vi "PSP-Nx-DM.vi"(0 "Cluster":cluster{"Button to Check":u16} {"Button to Check" items=["Start", "Select", "Up", "Down", "Left", "Right", "^", "[]", "X", "O", "L1", "L2", "L3", "R1", "R2", "R3"]}, 2 "NXT":T2={"error"={"status"=FALSE, "code"=0, "source"=""}, "address"="", "NXT #"=-1, "Show Error"=TRUE, "Connection"=4} {"Connection" items=["USB", "Bluetooth", "USB then Bluetooth", "Last Connection", "Preference"]}, 3 "Input Port":T3 items=["Port 1", "Port 2", "Port 3", "Port 4"]) -> (1 "output cluster":T1, 4 "NXT dup":T2={"error"={"status"=FALSE, "code"=0, "source"=""}, "address"="", "NXT #"=-1, "Show Error"=TRUE, "Connection"=4} {"Connection" items=["USB", "Bluetooth", "USB then Bluetooth", "Last Connection", "Preference"]})   [LabVIEW 2009]
uses:
  <vilib>/NXT/Block Support/NXT_InputPort.ctl
  <vilib>/NXT/Subs/LVHSConnector.ctl
  <vilib>/NXT/Block Support/HWPage.SensorType.ctl
  <vilib>/NXT/Block Support/HWPage.SensorMode.ctl
panel:
  # "mindsensors.com\nCopyright (c) 2009 by mindsensors.com\nEmail: info (<at>) mindsensors (<dot>) com\n\nThis program is free software. You can redistribute it and/or modify\nit under the terms of the GNU General Public License as published by\nthe Free Software Foundation; version 3 of the License.\nRead the license at: http://www.gnu.org/licenses/gpl.txt"
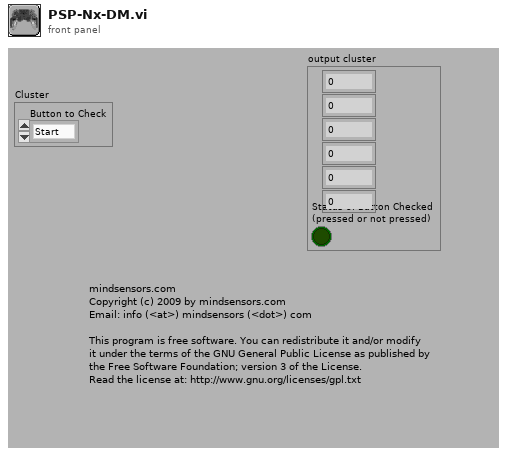
[diagram p1: front panel]
types:
  T1 = cluster{"left x":u8, "left y":u8, "right x":u8, "right y":u8, "button 1":u8, "button 2":u8, "Status of Button Checked\n(pressed or not pressed)":bool}
  T2 = typedef "LVHSConnector.ctl" = cluster{"error":errorcluster, "address":string, "NXT #":i32, "Show Error":bool, "Connection":u16}
  T3 = typedef "NXT_InputPort.ctl" = u8
  T4 = typedef "HWPage.SensorType.ctl" = u8
  T5 = typedef "HWPage.SensorMode.ctl" = u8
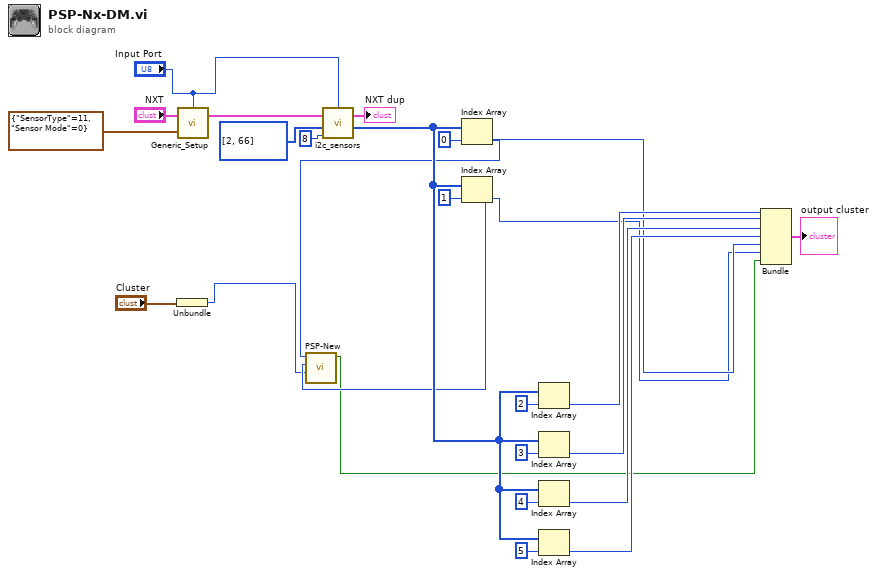
[diagram p0: block diagram]
diagram:
  n1 = Unbundle("Cluster") -> ("Button to Check"=w4:u16)
  n2 = call <vilib>:"Generic_Setup.vi"("Sensor Setup"=cluster{"SensorType":T4, "Sensor Mode":T5} {"SensorType"=11, "Sensor Mode"=0}, "NXT"="NXT", "Port"="Input Port") -> ("NXT"=w21:T2)  [unwired: 1 out]
  n3 = call <vilib>:"i2c_sensors.vi"("Return Length"=u8 8, "Bytes to Write"=u8[] [2, 66] ("Parameters"), "NXT"=w21, "Port"="Input Port") -> ("Bytes read"=w20:u8[], "NXT"=→"NXT dup":T2)  [unwired: 1 in, 1 out]
  n4 = Index Array(array=w20, index=0) -> (element=w7:u8)
  n5 = Index Array(array=w20, index=1) -> (element=w6:u8)
  n6 = call "PSP-New.vi"("Number"=w7, "Number 2"=w6, "Button to Check"=w4) -> ("Boolean"=w3:bool)  [unwired: 7 in]
  n7 = Index Array(array=w20, index=2) -> (element=w11:u8)
  n8 = Index Array(array=w20, index=3) -> (element=w10:u8)
  n9 = Index Array(array=w20, index=4) -> (element=w9:u8)
  n10 = Index Array(array=w20, index=5) -> (element=w8:u8)
  n11 = Bundle(w11, w10, w9, w8, w7, w6, "Boolean"=w3) -> (→"output cluster":cluster{u8, u8, u8, u8, u8, u8, "Boolean":bool})  [unwired: 1 in]
